vi "valve_fluigent.vi"(0 "MFCS_EZ_":T1, 1 "Delay_inlet(ms)":dbl, 2 "Delay_split(ms)":dbl, 3 "Delay (ms)":dbl, 5 "error in (no error)":errorcluster, 6 "inlet_high":dbl, 7 "split_high":dbl, 8 "inlet_low":dbl, 9 "split_low":dbl, 10 "inlet_ch":u8=1, 11 "split_ch":u8=1, 12 "Alpha_inlet (def: 5)":u8=5, 13 "Alpha_split (def: 5)":u8=5) -> (14 "MFCS_EZ out":T1, 19 "error out":errorcluster)   [LabVIEW 2018]
uses:
  <userlib>/Fluigent/Fluigent MFCS/FluigentMFCS_Full.llb/_mfcs_EZ_handle.ctl
  <userlib>/Fluigent/Fluigent MFCS/FluigentMFCS_Full.llb/MFCS_EZ Write Channel Pressure.vi
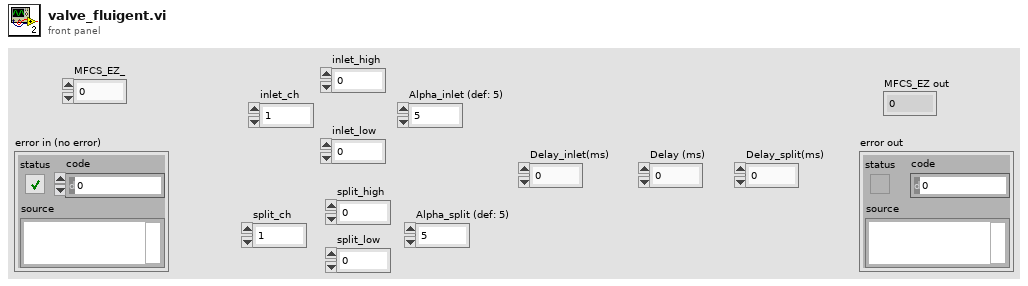
[diagram p1: front panel]
types:
  T1 = typedef "_mfcs_EZ_handle.ctl" = u64
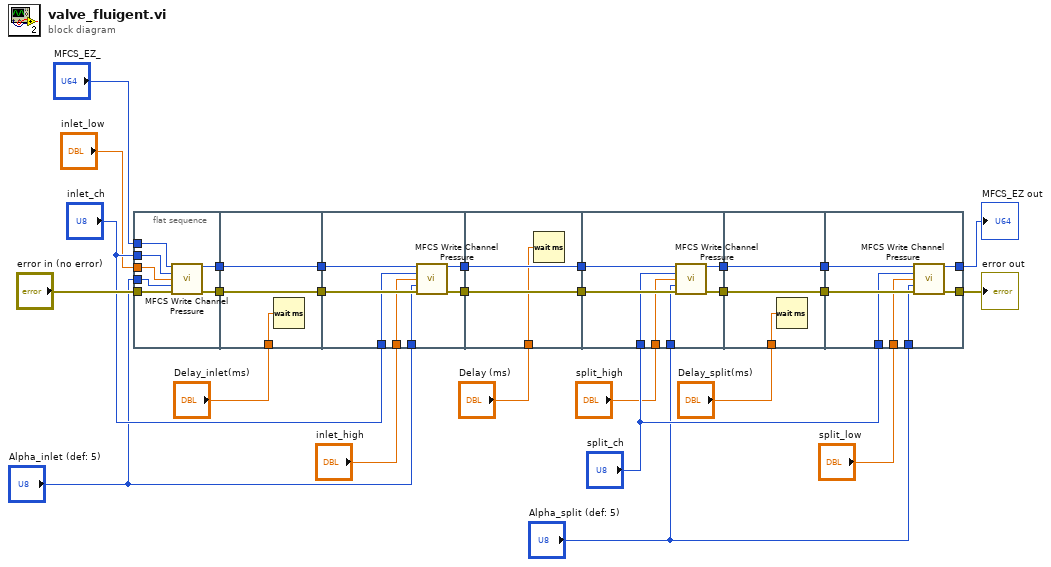
[diagram p0: block diagram]
diagram:
  n1 = flat-sequence {
    tunnel: [w34] -> w27
    tunnel: [w33] -> w26
    tunnel: "MFCS_EZ_" -> [w32]
    tunnel: "error in (no error)" -> [w31]
    tunnel: "inlet_ch" -> [w30]
    tunnel: "inlet_low" -> [w29]
    tunnel: "Alpha_inlet (def: 5)" -> [w28]
    tunnel: w27 -> [w37]
    tunnel: [w37] -> w25
    tunnel: w26 -> [w36]
    tunnel: [w36] -> w24
    tunnel: "Delay_inlet(ms)" -> [w35]
    tunnel: w25 -> [w44]
    tunnel: [w43] -> w23
    tunnel: w24 -> [w42]
    tunnel: [w41] -> w22
    tunnel: "inlet_ch" -> [w40]
    tunnel: "inlet_high" -> [w39]
    tunnel: "Alpha_inlet (def: 5)" -> [w38]
    tunnel: [w47] -> w21
    tunnel: w23 -> [w47]
    tunnel: [w46] -> w20
    tunnel: w22 -> [w46]
    tunnel: "Delay (ms)" -> [w45]
    tunnel: w21 -> [w54]
    tunnel: w20 -> [w53]
    tunnel: [w52] -> w19
    tunnel: [w51] -> w18
    tunnel: "split_ch" -> [w50]
    tunnel: "split_high" -> [w49]
    tunnel: "Alpha_split (def: 5)" -> [w48]
    tunnel: "Delay_split(ms)" -> [w57]
    tunnel: [w56] -> w17
    tunnel: w19 -> [w56]
    tunnel: [w55] -> w16
    tunnel: w18 -> [w55]
    tunnel: w17 -> [w64]
    tunnel: w16 -> [w63]
    tunnel: "split_ch" -> [w62]
    tunnel: "split_low" -> [w61]
    tunnel: "Alpha_split (def: 5)" -> [w60]
    tunnel: [w59] -> w2
    tunnel: [w58] -> w1
    frame #0 {
      n2 = call-poly <userlib>:"MFCS Write Channel Pressure.vi"("MFCS_EZ"=w32, "Channel Number (default=1)"=w30, "Pressure (mBar)"=w29, "Alpha (default=5)"=w28, "error in (no error)"=w31) -> ("MFCS_EZ out"=w34:T1, "error out"=w33:errorcluster)  [unwired: 9 in]
    }
    frame #1 {
      n3 = Wait (ms)(milliseconds to wait=w35) -> ()  [unwired: 1 out]
    }
    frame #2 {
      n4 = call-poly <userlib>:"MFCS Write Channel Pressure.vi"("MFCS_EZ"=w44, "Channel Number (default=1)"=w40, "Pressure (mBar)"=w39, "Alpha (default=5)"=w38, "error in (no error)"=w42) -> ("MFCS_EZ out"=w43:T1, "error out"=w41:errorcluster)  [unwired: 9 in]
    }
    frame #3 {
      n5 = Wait (ms)(milliseconds to wait=w45) -> ()  [unwired: 1 out]
    }
    frame #4 {
      n6 = call-poly <userlib>:"MFCS Write Channel Pressure.vi"("MFCS_EZ"=w54, "Channel Number (default=1)"=w50, "Pressure (mBar)"=w49, "Alpha (default=5)"=w48, "error in (no error)"=w53) -> ("MFCS_EZ out"=w52:T1, "error out"=w51:errorcluster)  [unwired: 9 in]
    }
    frame #5 {
      n7 = Wait (ms)(milliseconds to wait=w57) -> ()  [unwired: 1 out]
    }
    frame #6 {
      n8 = call-poly <userlib>:"MFCS Write Channel Pressure.vi"("MFCS_EZ"=w64, "Channel Number (default=1)"=w62, "Pressure (mBar)"=w61, "Alpha (default=5)"=w60, "error in (no error)"=w63) -> ("MFCS_EZ out"=w59:T1, "error out"=w58:errorcluster)  [unwired: 9 in]
    }
  }
  "MFCS_EZ out" <- w2
  "error out" <- w1
